vi "Lift speed controller.vi"(6 "Speed in":dbl=1.0, 7 "Distance decel":dbl, 9 "Position after lift is done moving":dbl, 10 "Are we moving?":bool, 11 "Distance accel":dbl) -> (3 "Speed out":dbl)   [LabVIEW 2014]
uses:
  Begin/Global Variables.vi
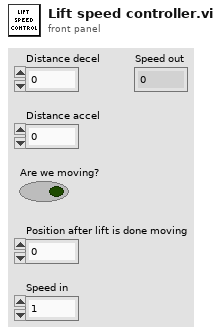
[diagram p1: front panel]
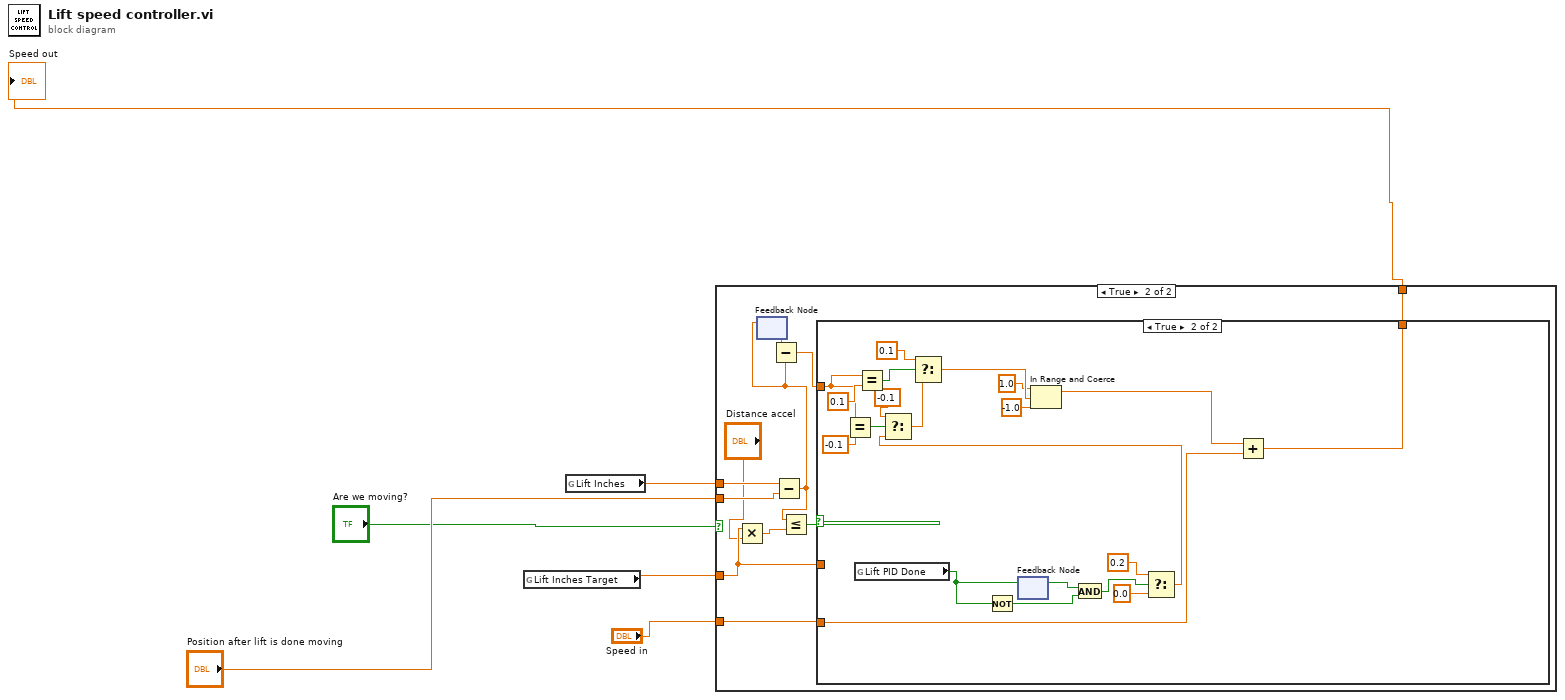
[diagram p0: block diagram]
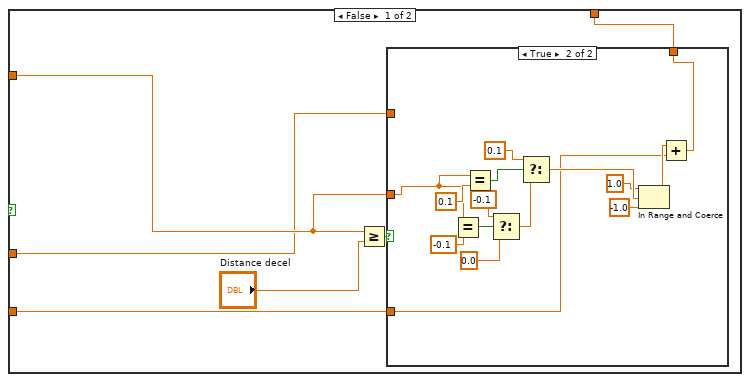
[diagram p3: hidden frame]
diagram:
  n1 = global read "Global Variables.vi" "Lift Inches Target"() -> (w2:dbl)
  n2 = global read "Global Variables.vi" "Lift Inches"() -> (w6:dbl)
  n3 = case shown="True" "Are we moving?" {
    tunnel: "Speed in" -> [w7 w16]
    tunnel: [w7 w17] -> w3
    tunnel: w2 -> [_ w12]
    tunnel: w6 -> [_ w15]
    tunnel: "Position after lift is done moving" -> [_ w14]
    frame False {
    }
    frame True {
      n4 = Multiply(x=w12, y="Distance accel") -> (x*y=w13:dbl)
      n5 = feedback #1() -> (w10:dbl)  [unwired: 1 in]
      n6 = Subtract(x=w15, y=w14) -> (x-y=w9:dbl)
      n7 = feedback-in #1(w9) -> ()
      n8 = Subtract(x=w10, y=w9) -> (x-y=w8:dbl)
      n9 = Less Or Equal?(x=w9, y=w13) -> (x <= y?=w18:bool)
      n10 = case shown="True" w18 {
        tunnel: w8 -> [w23 w49]
        tunnel: [w22 w42] -> w17
        tunnel: w16 -> [w21 w41]
        tunnel: w12 -> [w20 _]
        frame False {
          n11 = Greater Or Equal?(x=w23, y="Distance decel") -> (x >= y?=w24:bool)
          n12 = case shown="True" w24 {
            tunnel: w23 -> [_ w30]
            tunnel: w20 -> [_ _]
            tunnel: [w25 w26] -> w22
            tunnel: w21 -> [w25 w27]
            frame False {
            }
            frame True {
              n13 = Equal?(x=w30, y=-0.1) -> (x = y?=w33:bool)
              n14 = Equal?(x=w30, y=0.1) -> (x = y?=w39:bool)
              n15 = Select(t=-0.1, s=w33, f=0.0) -> (s? t:f=w32:dbl)
              n16 = Select(t=0.1, s=w39, f=w32) -> (s? t:f=w37:dbl)
              n17 = In Range and Coerce(upper limit=1.0, x=w37, lower limit=-1.0) -> (coerced(x)=w28:dbl)  [unwired: 1 out]
              n18 = Add(x=w28, y=w27) -> (x+y=w26:dbl)
            }
          }
        }
        frame True {
          n19 = Equal?(x=w49, y=-0.1) -> (x = y?=w47:bool)
          n20 = global read "Global Variables.vi" "Lift PID Done"() -> (w58:bool)
          n21 = Equal?(x=w49, y=0.1) -> (x = y?=w54:bool)
          n22 = Not(x=w58) -> (.not. x?=w57:bool)
          n23 = feedback #2() -> (w59:bool)  [unwired: 1 in]
          n24 = feedback-in #2(w58) -> ()
          n25 = And(x=w59, y=w57) -> (x .and. y?=w56:bool)
          n26 = Select(t=0.2, s=w56, f=0.0) -> (s? t:f=w46:dbl)
          n27 = Select(t=-0.1, s=w47, f=w46) -> (s? t:f=w45:dbl)
          n28 = Select(t=0.1, s=w54, f=w45) -> (s? t:f=w52:dbl)
          n29 = In Range and Coerce(upper limit=1.0, x=w52, lower limit=-1.0) -> (coerced(x)=w43:dbl)  [unwired: 1 out]
          n30 = Add(x=w43, y=w41) -> (x+y=w42:dbl)
        }
      }
    }
  }
  "Speed out" <- w3
